vi "Panel Resize.vi"(0 "Width":i16, 1 "Height":i16, 3 "error in (no error)":errorcluster, 4 "reference":refnum<vi>) -> (10 "error out":errorcluster)   [LabVIEW 2018]
uses:
  <vilib>/Utility/miscctls.llb/LVPointTypeDef.ctl
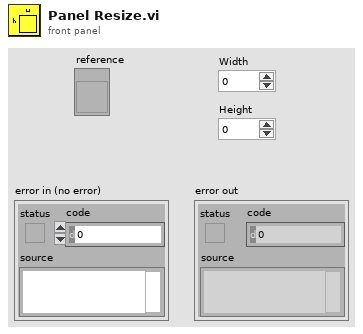
[diagram p1: front panel]
types:
  T1 = typedef "LVPointTypeDef.ctl" = cluster{"Horizontal":i16, "Vertical":i16}
  T2 = typedef "LVRectTypeDef.ctl" = cluster{"Left":i16, "Top":i16, "Right":i16, "Bottom":i16}
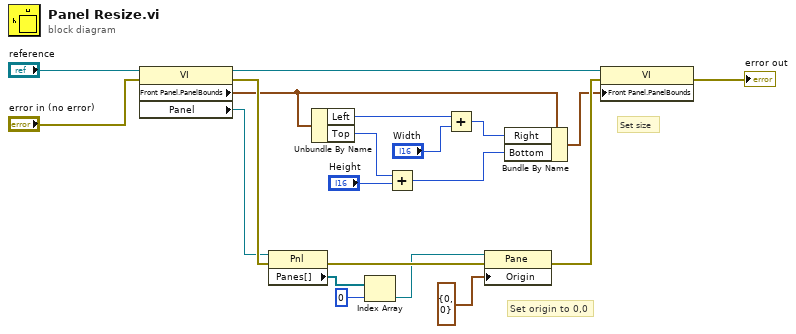
[diagram p0: block diagram]
diagram:
  # "Set origin to 0,0"
  # "Set size"
  n1 = property class="VI"(reference="reference", error in="error in (no error)") -> (reference out=w14:refnum<vi>, error out=w18:errorcluster, "Front Panel.PanelBounds"=w6:T2, "Panel"=w5:refnum<vi>)
  n2 = property class="Pnl"(reference=w5, error in=w18) -> (error out=w17:errorcluster, "Panes[]"=w4:refnum<vi>[])  [unwired: 1 out]
  n3 = Unbundle By Name(w6) -> ("Left"=w7:i16, "Top"=w11:i16)
  n4 = Index Array(array=w4, index=0) -> (element=w2:refnum<vi>)
  n5 = Add(x=w11, y="Height") -> (x+y=w10:i16)
  n6 = Add(x=w7, y="Width") -> (x+y=w8:i16)
  n7 = property class="Pane"(reference=w2, error in=w17, "Origin"=T1 {"Horizontal"=0, "Vertical"=0}) -> (error out=w19:errorcluster)  [unwired: 1 out]
  n8 = Bundle By Name(cluster=w6, "Right"=w8, "Bottom"=w10) -> (w15:T2)
  n9 = property class="VI"(reference=w14, error in=w19, "Front Panel.PanelBounds"=w15) -> (error out=→"error out":errorcluster)  [unwired: 1 out]
